vi "PhidgetNet_setServerPassword.vi"(8 "error in":errorcluster, 10 "Password":string, 11 "Server Name":string) -> (0 "error out":errorcluster)   [LabVIEW 2012, in "Phidget Common.lvlib"]
doc: "${SetServerPassword:Header}"
uses:
  <instrlib>/Phidgets/Phidget Common/Phidget Common.lvlib
  phidget22.dll
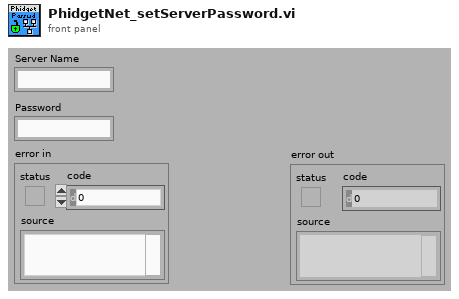
[diagram p1: front panel]
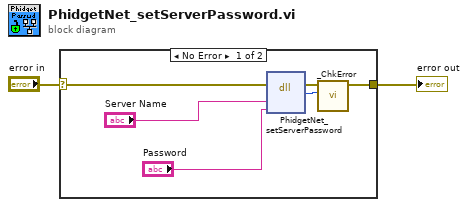
[diagram p0: block diagram]
diagram:
  n1 = case shown="No Error" "error in" {
    selector: "error in" -> [w6 w9]
    tunnel: [w4 w9] -> w1
    frame No Error {
      n2 = dll-call lib="phidget22.dll" fn="PhidgetNet_setServerPassword"(error in=w6, "srvname"="Server Name", "passwd"="Password") -> (error out=w5:errorcluster, "return type"=w8:i32)  [unwired: 4 in, 1 out]
      n3 = call <instrlib>:"_ChkError.vi"("Return Code"=w8, "error in (no error)"=w5) -> ("error out"=w4:errorcluster)  [unwired: 9 in]
    }
    frame Error {
    }
  }
  "error out" <- w1
